vi "LINX_-_BallAndBeam_v8.vi"() -> ()   [LabVIEW 2018]
doc: "Manually blink and LED attached to a digital output channel of a LINX device by clicking and LED control in LabVIEW."
uses:
  <vilib>/addons/control/pid/pid.llb/PID Structure.ctl
  <vilib>/addons/control/pid/pid.llb/PID Time Unit.ctl
  <vilib>/addons/control/pid/pid.llb/PID Gain Unit.ctl
  <vilib>/MakerHub/LINX/Public/Peripherals/Analog/Analog Read 1 Chan.vi
  <vilib>/MakerHub/LINX/Public/Peripherals/Analog/Analog Read N Chans.vi
  <vilib>/MakerHub/LINX/Private/Local IO/LinxAnalogRead.vi
  <vilib>/MakerHub/LINX/Public/Utilities/Check Channel.vi
  <vilib>/MakerHub/LINX/Public/Utilities/Open Serial.vi
  <vilib>/MakerHub/LINX/Public/Sensors/Motion/Servo/Servo Open One Channel.vi
  <vilib>/addons/control/pid/pid.llb/PID Structure Conversion (DBL).vi
  <vilib>/MakerHub/LINX/Private/Utilties/Generate Error.vi
  <vilib>/addons/control/pid/pid.llb/PID Advanced (DBL).vi
  <vilib>/MakerHub/LINX/Public/Sensors/Motion/Servo/Servo Set Pulse Width One Channel.vi
  <vilib>/MakerHub/LINX/Public/Sensors/Motion/Servo/Servo Close One Channel.vi
  <vilib>/MakerHub/LINX/LMH-LINX.lvlib
  <vilib>/MakerHub/LINX/Public/Sensors/Motion/Servo/Servo.lvlib
  <vilib>/addons/control/pid/NI_PID_pid.lvlib
  <vilib>/ptbypt/NI_PtbyPt.lvlib
panel:
  in  "Sensor pin":i32
  in  "Servo pin":u32
  out "Slide":dbl(slide) scale=0.0..60.0
  in  "PID (dt)":dbl
  out "PID (dt)":dbl
  in  "Proportional Unit":T1 items=["Gain (Kc)", "Band (PB)"]
  in  "Derivative Unit":T2 items=["min", "s"]
  in  "Integral Unit":T2 items=["min", "s"]
  in  "PID Topology":T3 items=["Academic (Standard)", "Parallel", "Series"]
  in  "Derivative":dbl format="%#.3g"
  in  "Integral":dbl=0.008 format="%#.3g"
  in  "Proportional":dbl=5.0 format="%#.10f"
  in  "Initialize":bool
  out "Manual setpoint 2":dbl(slide) scale=0.0..60.0
  out "Waveform Chart":cluster{"Setpoint":dbl, dbl, "servo":dbl}(graph)
  in  "setpoint range":cluster{"setpoint high":dbl, "setpoint low":dbl}={"setpoint high"=60.0, "setpoint low"=0.0} {"setpoint high" min=0.0 max=60.0 format="%.2f"; "setpoint low" min=0.0 max=60.0 format="%.2f"}
  out "Lamp":bool
  out "output":dbl format="%.1f"
  in  "output range":cluster{"output high":dbl, "output low":dbl}={"output high"=100.0, "output low"=0.0} {"output low" min=0.0 max=2500.0 format="%.2f"; "output high" min=0.0 max=2500.0 format="%.2f"}
  out "Distance":dbl format="%.1g"
  in  "Setpoint":dbl
  in  "Manual":bool
  in  "Manual setpoint":dbl(slide) scale=0.0..100.0
  out "Loop Rate (Hz)":u32
  in  "Serial Port":refnum<visa-resource-name>
  in  "Stop Button":bool
  # "Within 1 cm of S.P.\nPID Gain"
  # "Working variable values:"
  # "Setpoint"
  # "Distance"
  # "LINX Device Settings"
  # "Manual override servo"
  # "PID output\nPID Gain"
  # "PID (dt)                  = 0.02\n\nAveraging distance = 10\n\nAveraging servo       = 10\n\nOutput high            = 70,0\nOutput low              = 0,00\n\nSetpoint high           = 60,0\nSetpoint low            = 0,0\n\nProportional             = 1,0\nIntegral                   = 1,3s\nDerivative               = 1,51s"
  # "Graph\nPID Gain"
  # "Output range\nPID Gain"
  # "-\nPID Gain"
  # "Setpoint range\nSetpoint range\nPID Gain"
  # "Ball and Beam"
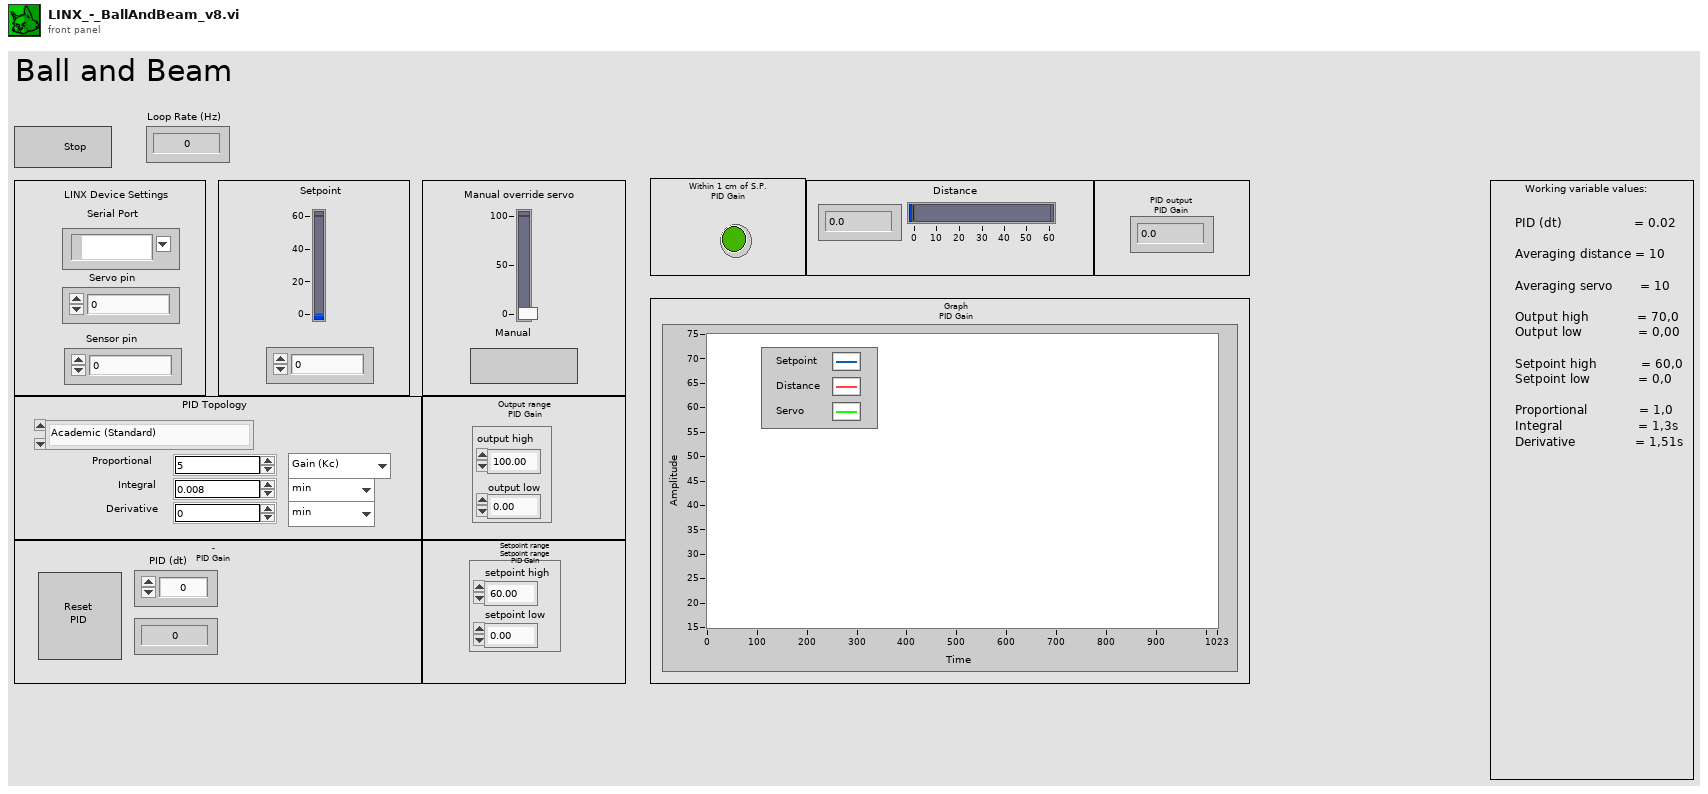
[diagram p1: front panel]
types:
  T1 = typedef "NI_PID_pid.lvlib/PID Gain Unit.ctl" = u16
  T2 = typedef "NI_PID_pid.lvlib/PID Time Unit.ctl" = u16
  T3 = typedef "NI_PID_pid.lvlib/PID Structure.ctl" = u16
  T4 = typedef "LMH-LINX.lvlib/LINX Ref.ctl" = cluster{"IO":T5, "Interface":T6, "LINX Device Config":T7}
  T5 = typedef "LMH-LINX.lvlib/Platform.ctl" = enum16{"Remote", "Local"}
  T6 = typedef "LMH-LINX.lvlib/Interface.ctl" = enum16{"Serial", "TCP"}
  T7 = typedef "LMH-LINX.lvlib/Device.lvlib/LINX Device Config.ctl" = cluster{"Interface":T6, "COM Port":refnum<visa-resource-name>, "TCP Configuration":T8, "Device Family":u8, "Device ID":u8, "Device Name":string, "TCP Ref":refnum<k5>, "Channels":T9}
  T8 = typedef "LMH-LINX.lvlib/Device.lvlib/TCP Config.ctl" = cluster{"IP Address":string, "Port":u16}
  T9 = typedef "LMH-LINX.lvlib/Channels.ctl" = cluster{"DI":u8[], "DO":u8[], "AI":u8[], "AO":u8[], "PWM":u8[], "QE":u8[], "UART":u8[], "I2C 2":u8[], "SPI":u8[], "CAN":u8[], "Servo":u8[], "AI Ref (V)":dbl, "AI Resolution (Bits)":u8, "AO Ref (V)":dbl, "AO Resolution (Bits)":u8}
  T10 = cluster{"proportional gain (Kc)":dbl, "integral time (Ti, min)":dbl, "derivative time (Td, min)":dbl}
  T11 = cluster{"Setpoint":dbl, "dist":dbl, "output":dbl}
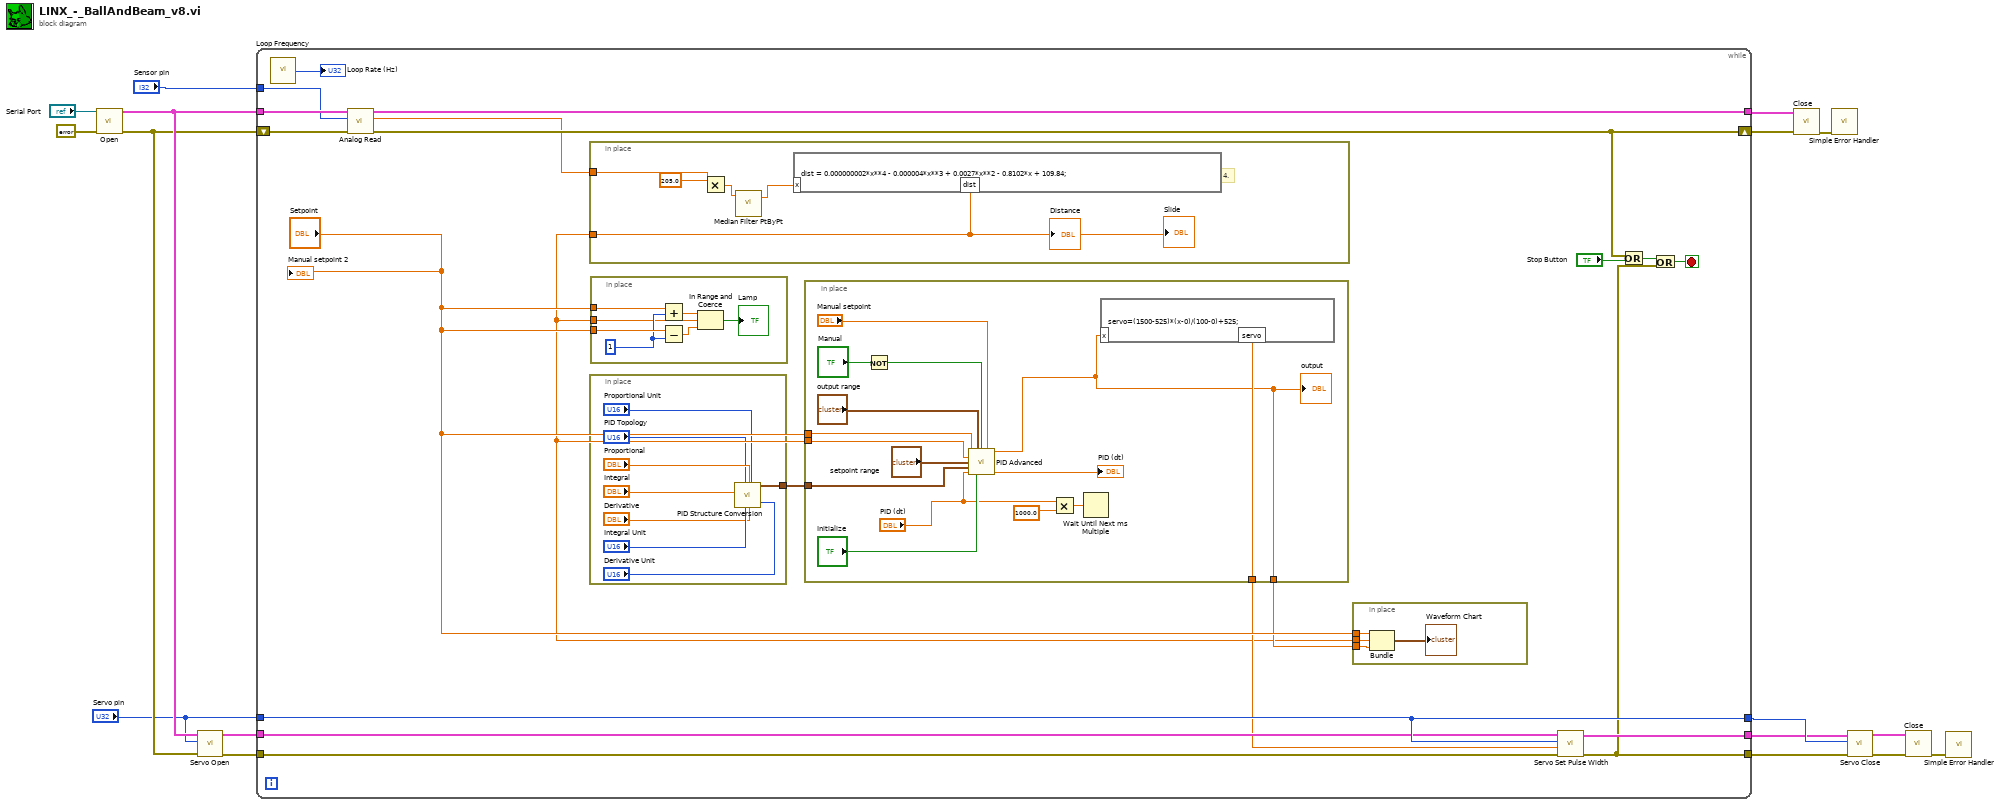
[diagram p0: block diagram]
diagram:
  # "4."
  # "3."
  n1 = call-poly <vilib>:"Open.vi"("Error In"=errorcluster {"status"=FALSE, "code"=0, "source"=""}, "Serial Port"="Serial Port") -> ("Error Out"=w14:errorcluster, "LINX Resource"=w15:T4)  [unwired: 7 in, 1 out]
  n2 = call-poly <vilib>:"Servo Open.vi"("Error In"=w14, "Servo Channel"="Servo pin", "LINX Resource"=w15) -> ("Error Out"=w9:errorcluster, "LINX Resource"=w10:T4)  [unwired: 7 in]
  n3 = while {
    tunnel: w15 -> [w35]
    tunnel: [w29] -> w7
    shift-right: [w28] -> w6
    shift-left: w14 -> [w34]
    tunnel: [w25] -> w3
    tunnel: [w33] -> w4
    tunnel: [w32] -> w5
    tunnel: "Servo pin" -> [w32]
    tunnel: w10 -> [w31]
    tunnel: w9 -> [w30]
    tunnel: "Sensor pin" -> [w18]
    stop <- w27 stop-if-true
    n4 = call <vilib>:"Loop Frequency.vi"() -> ("Loop Rate (Hz)"=→"Loop Rate (Hz)":u32)
    n5 = call-poly <vilib>:"Analog Read.vi"("Error In"=w34, "Analog Channel"=w18, "LINX Resource"=w35) -> ("Error Out"=w28:errorcluster, "Voltage"=w22:dbl, "LINX Resource"=w29:T4)  [unwired: 5 in, 1 out]
    n6 = in-place {
      in-place-border: [w67] -> w19
      in-place-border: w22 -> [w68]
      n7 = Multiply(x=205.0, y=w68) -> (x*y=w66:dbl)
      n8 = call <vilib>:"Median Filter PtByPt.vi"("x"=w66) -> ("Filtered x"=w65:dbl)  [unwired: 3 in, 1 out]
      n9 = formula code="dist = 0.000000002*x**4 - 0.000004*x**3 + 0.0027*x**2 - 0.8102*x + 109.84;"("x"=w65) -> ("dist"=w67:dbl)
      "Distance" <- w67
      "Slide" <- w67
    }
    n10 = in-place {
      in-place-border: [w57] -> w24
      n11 = call-poly <vilib>:"PID Structure Conversion.vi"("derivative unit"="Derivative Unit", "proportional unit"="Proportional Unit", "integral unit"="Integral Unit", "PID structure"="PID Topology", "derivative"="Derivative", "integral"="Integral", "proportional"="Proportional") -> ("PID gains"=w57:T10)  [unwired: 4 in]
    }
    n12 = in-place {
      in-place-border: "Setpoint" -> [w74]
      in-place-border: "Setpoint" -> [w73]
      in-place-border: w19 -> [w70]
      w72 = 1
      n13 = Add(x=w73, y=w72) -> (x+y=w76:dbl)
      n14 = Subtract(x=w74, y=w72) -> (x-y=w71:dbl)
      n15 = In Range and Coerce(upper limit=w76, x=w70, lower limit=w71) -> (In Range?=→"Lamp":bool)  [unwired: 1 out]
    }
    n16 = in-place {
      in-place-border: w24 -> [w50]
      in-place-border: "Setpoint" -> [w46]
      in-place-border: w19 -> [w47]
      in-place-border: [w43] -> w21
      in-place-border: [w42] -> w20
      n17 = Not(x="Manual") -> (.not. x?=w52:bool)
      n18 = call-poly <vilib>:"PID Advanced.vi"("setpoint"=w46, "output range"="output range", "auto? (T)"=w52, "manual control"="Manual setpoint", "process variable"=w47, "setpoint range"="setpoint range", "PID gains"=w50, "dt (s)"="PID (dt)", "reinitialize? (F)"="Initialize") -> ("output"=w42:dbl, "dt out (s)"=→"PID (dt)":dbl)  [unwired: 5 in]
      "output" <- w42
      n19 = Multiply(x="PID (dt)", y=1000.0) -> (x*y=w48:dbl)
      n20 = Wait Until Next ms Multiple(millisecond multiple=w48) -> ()  [unwired: 1 out]
      n21 = formula code="servo=(1500-525)*(x-0)/(100-0)+525;"("x"=w42) -> ("servo"=w43:dbl)
    }
    n22 = in-place {
      in-place-border: "Setpoint" -> [w40]
      in-place-border: w19 -> [w39]
      in-place-border: w20 -> [w38]
      n23 = Bundle("Setpoint"=w40, "dist"=w39, "output"=w38) -> (→"Waveform Chart":T11)  [unwired: 1 in]
    }
    n24 = call-poly <vilib>:"Servo Set Pulse Width.vi"("Error In"=w30, "Pulse Width (uS)"=w21, "Servo Channel"=w32, "LINX Resource"=w31) -> ("Error Out"=w25:errorcluster, "LINX Resource"=w33:T4)  [unwired: 6 in]
    n25 = Or(x=w28, y="Stop Button") -> (x .or. y?=w26:bool)
    n26 = Or(x=w26, y=w25) -> (x .or. y?=w27:bool)
    "Manual setpoint 2" <- "Setpoint"
  }
  n27 = call <vilib>:"Close.vi"("Error In"=w6, "LINX Resource"=w7) -> ("Error Out"=w8:errorcluster)  [unwired: 9 in]
  n28 = call <vilib>:"Simple Error Handler.vi"("error in (no error)"=w8) -> ()  [unwired: 4 in, 5 out]
  n29 = call-poly <vilib>:"Servo Close.vi"("Error In"=w3, "Servo Channel"=w5, "LINX Resource"=w4) -> ("Error Out"=w13:errorcluster, "LINX Resource"=w12:T4)  [unwired: 7 in]
  n30 = call <vilib>:"Close.vi"("Error In"=w13, "LINX Resource"=w12) -> ("Error Out"=w11:errorcluster)  [unwired: 9 in]
  n31 = call <vilib>:"Simple Error Handler.vi"("error in (no error)"=w11) -> ()  [unwired: 4 in, 5 out]
